vi "Build Dqmh Module Relationship Graph.vi"(4 "Used Requests With Reply":T1[](array[typedef]), 6 "Request With Reply Links Info":T2[](array[typedef]), 7 "Module Name":string, 8 "Used Requests":T1[](array[typedef]), 9 "Registred Broadcast":T3[](array[typedef]), 10 "Broadcas Links Info":T2[](array[typedef]), 11 "Request Links Info":T2[](array[typedef])) -> (3 "Graph":string)   [LabVIEW 2021, in "TAF Proj Document Type.lvlib" / "Dqmh Module.lvclass"]
uses:
  <vilib>/Wovalab/AntiDoc/Document Type/Add-ons/LabVIEW TAF Project/Dqmh Module/Dqmh Module.lvclass
  <vilib>/Wovalab/AntiDoc/Document Type/Add-ons/LabVIEW TAF Project/Dqmh Module/Event Callers--cluster.ctl
  <vilib>/Wovalab/AntiDoc/Document Type/Add-ons/LabVIEW TAF Project/Dqmh Module/Module Broadcast Registred--cluster.ctl
  <vilib>/Wovalab/AntiDoc/Document Type/Add-ons/LabVIEW TAF Project/Dqmh Module/Requests Used By Module--cluster.ctl
  <vilib>/Wovalab/AntiDoc/GraphBuilder/Renderer/Graphviz/Graphviz.lvclass
  C:/Program Files (x86)/National Instruments/LabVIEW 2021/vi.lib/Wovalab/AntiDoc/GraphBuilder/Renderer/Renderer.lvclass
  <vilib>/Wovalab/AntiDoc/GraphBuilder/Graph/Graph.lvclass
  <vilib>/Wovalab/AntiDoc/GraphBuilder/Shapes/Edge/Graphviz/Graphviz Edge Shape.lvclass
  <vilib>/Wovalab/AntiDoc/GraphBuilder/Shapes/Edge/Graphviz/Shape.ctl
  <vilib>/Wovalab/AntiDoc/GraphBuilder/Shapes/Edge/Graphviz/Colors.ctl
  <vilib>/Wovalab/AntiDoc/GraphBuilder/Shapes/Node/Graphviz/Colors.ctl
  <vilib>/Wovalab/AntiDoc/GraphBuilder/Shapes/Node/Graphviz/Shape.ctl
  <vilib>/Wovalab/AntiDoc/GraphBuilder/Renderer/Graphviz/Specific Node Shape Def.ctl
  <vilib>/Wovalab/AntiDoc/GraphBuilder/Shapes/Node/Graphviz/Graphviz Node Shape.lvclass
  <vilib>/Wovalab/AntiDoc/GraphBuilder/Node/Node.lvclass
  <vilib>/Wovalab/AntiDoc/Document Type/Add-ons/LabVIEW TAF Project/Dqmh Module/Link Type--enum.ctl
  <vilib>/Wovalab/AntiDoc/GraphBuilder/Renderer/Graphviz/Graph Direction.ctl
  <vilib>/Wovalab/AntiDoc/Document Type/Add-ons/LabVIEW TAF Project/TAF Proj Document Type.lvlib
  <vilib>/Wovalab/AntiDoc/Utilities/Utilities.lvlib
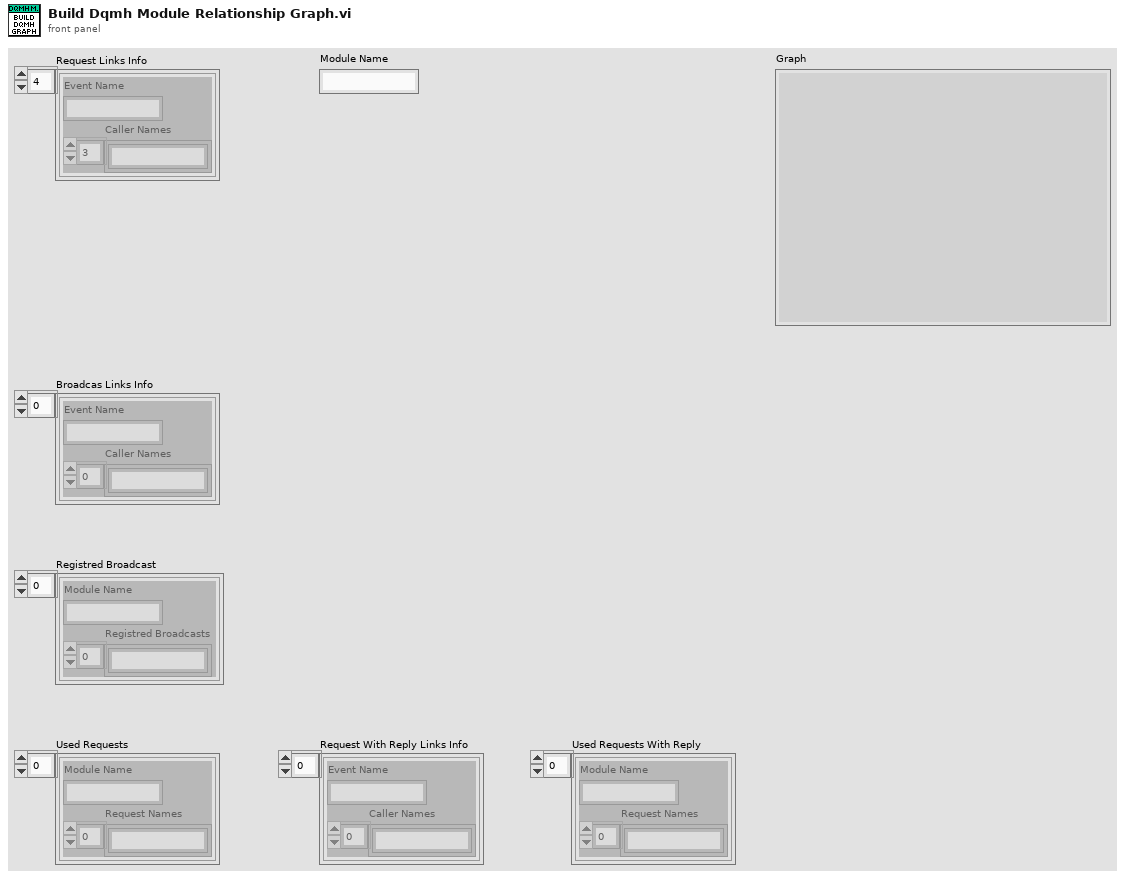
[diagram p1: front panel]
types:
  T1 = typedef "TAF Proj Document Type.lvlib/Dqmh Module.lvclass/Requests Used By Module--cluster.ctl" = cluster{"Module Name":string, "Request Names":string[]}
  T2 = typedef "TAF Proj Document Type.lvlib/Dqmh Module.lvclass/Event Callers--cluster.ctl" = cluster{"Event Name":string, "Caller Names":string[]}
  T3 = typedef "TAF Proj Document Type.lvlib/Dqmh Module.lvclass/Module Broadcast Registred--cluster.ctl" = cluster{"Module Name":string, "Registred Broadcasts":string[]}
  T4 = typedef "TAF Proj Document Type.lvlib/Dqmh Module.lvclass/Link Type--enum.ctl" = enum16{"Request", "Request With Reply", "Broadcast", "Registred Broadcast", "Used Requests", "Used Requests With Reply"}
  T5 = typedef "GraphBuilder.lvlib/Graphviz.lvclass/Graph Direction.ctl" = enum16{"Top to Bottom", "Left To Right", "Bottom to Top", "Right to Left"}
  T6 = typedef "GraphBuilder.lvlib/Graphviz Node Shape.lvclass/Colors.ctl" = enum16{"aliceblue", "antiquewhite", "aqua", "aquamarine", "azure", "beige", "bisque", "black", "blanchedalmond", "blue", "blueviolet", "brown", "burlywood", "cadetblue", "chartreuse", "chocolate", "coral", "cornflowerblue", "cornsilk", "crimson", "cyan", "darkblue", "darkcyan", "darkgoldenrod", "darkgray", "darkgreen", "darkgrey", "darkkhaki", "darkmagenta", "darkolivegreen", "darkorange", "darkorchid", "darkred", "darksalmon", "darkseagreen", "darkslateblue", "darkslategray", "darkslategrey", "darkturquoise", "darkviolet", "deeppink", "deepskyblue", "dimgray", "dimgrey", "dodgerblue", "firebrick", "floralwhite", "forestgreen", "fuchsia", "gainsboro", "ghostwhite", "gold", "goldenrod", "gray", "green", "greenyellow", "grey", "honeydew", "hotpink", "indianred", "indigo", "ivory", "khaki", "lavender", "lavenderblush", "lawngreen", "lemonchiffon", "lightblue", "lightcoral", "lightcyan", "lightgoldenrodyellow", "lightgray", "lightgreen", "lightgrey", "lightpink", "lightsalmon", "lightseagreen", "lightskyblue", "lightslategray", "lightslategrey", "lightsteelblue", "lightyellow", "lime", "limegreen", "linen", "magenta", "maroon", "mediumaquamarine", "mediumblue", "mediumorchid", "mediumpurple", "mediumseagreen", "mediumslateblue", "mediumspringgreen", "mediumturquoise", "mediumvioletred", "midnightblue", "mintcream", "mistyrose", "moccasin", "navajowhite", "navy", "oldlace", "olive", "olivedrab", "orange", "orangered", "orchid", "palegoldenrod", "palegreen", "paleturquoise", "palevioletred", "papayawhip", "peachpuff", "peru", "pink", "plum", "powderblue", "purple", "red", "rosybrown", "royalblue", "saddlebrown", "salmon", "sandybrown", "seagreen", "seashell", "sienna", "silver", "skyblue", "slateblue", "slategray", "slategrey", "snow", "springgreen", "steelblue", "tan", "teal", "thistle", "tomato", "turquoise", "violet", "wheat", "white", "whitesmoke", "yellow", "yellowgreen"}
  T7 = typedef "GraphBuilder.lvlib/Graphviz.lvclass/Specific Node Shape Def.ctl" = cluster{"Node ID":string, "Graphviz Node Shape":refnum<class "Graphviz Node Shape.lvclass">}
  T8 = typedef "GraphBuilder.lvlib/Graphviz Node Shape.lvclass/Shape.ctl" = enum16{"box", "polygon", "ellipse", "oval", "circle", "point", "egg", "triangle", "plaintext", "plain", "diamond", "trapezium", "parallelogram", "house", "pentagon", "hexagon", "septagon", "octagon", "doublecircle", "doubleoctagon", "tripleoctagon", "invtriangle", "invtrapezium", "invhouse", "Mdiamond", "Msquare", "Mcircle", "rect", "rectangle", "square", "star", "none", "underline", "cylinder", "note", "tab", "folder", "box3D", "component", "promoter", "cds", "terminator", "utr", "primersite", "restrictionsite", "fivepoverhang", "threepoverhang", "noverhang", "assembly", "signature", "insulator", "ribosite", "rnastab", "proteasesite", "proteinstab", "rpromoter", "rarrow", "larrow", "lpromoter"}
  T9 = typedef "GraphBuilder.lvlib/Graphviz Edge Shape.lvclass/Colors.ctl" = enum16{"aliceblue", "antiquewhite", "aqua", "aquamarine", "azure", "beige", "bisque", "black", "blanchedalmond", "blue", "blueviolet", "brown", "burlywood", "cadetblue", "chartreuse", "chocolate", "coral", "cornflowerblue", "cornsilk", "crimson", "cyan", "darkblue", "darkcyan", "darkgoldenrod", "darkgray", "darkgreen", "darkgrey", "darkkhaki", "darkmagenta", "darkolivegreen", "darkorange", "darkorchid", "darkred", "darksalmon", "darkseagreen", "darkslateblue", "darkslategray", "darkslategrey", "darkturquoise", "darkviolet", "deeppink", "deepskyblue", "dimgray", "dimgrey", "dodgerblue", "firebrick", "floralwhite", "forestgreen", "fuchsia", "gainsboro", "ghostwhite", "gold", "goldenrod", "gray", "green", "greenyellow", "grey", "honeydew", "hotpink", "indianred", "indigo", "ivory", "khaki", "lavender", "lavenderblush", "lawngreen", "lemonchiffon", "lightblue", "lightcoral", "lightcyan", "lightgoldenrodyellow", "lightgray", "lightgreen", "lightgrey", "lightpink", "lightsalmon", "lightseagreen", "lightskyblue", "lightslategray", "lightslategrey", "lightsteelblue", "lightyellow", "lime", "limegreen", "linen", "magenta", "maroon", "mediumaquamarine", "mediumblue", "mediumorchid", "mediumpurple", "mediumseagreen", "mediumslateblue", "mediumspringgreen", "mediumturquoise", "mediumvioletred", "midnightblue", "mintcream", "mistyrose", "moccasin", "navajowhite", "navy", "oldlace", "olive", "olivedrab", "orange", "orangered", "orchid", "palegoldenrod", "palegreen", "paleturquoise", "palevioletred", "papayawhip", "peachpuff", "peru", "pink", "plum", "powderblue", "purple", "red", "rosybrown", "royalblue", "saddlebrown", "salmon", "sandybrown", "seagreen", "seashell", "sienna", "silver", "skyblue", "slateblue", "slategray", "slategrey", "snow", "springgreen", "steelblue", "tan", "teal", "thistle", "tomato", "turquoise", "violet", "wheat", "white", "whitesmoke", "yellow", "yellowgreen"}
  T10 = typedef "GraphBuilder.lvlib/Graphviz Edge Shape.lvclass/Shape.ctl" = enum16{"box", "lbox", "rbox", "obox", "olbox", "orbox", "crow", "lcrow", "rcrow", "diamond", "ldiamond", "rdiamond", "odiamond", "oldiamond", "ordiamond", "dot", "odot", "inv", "linv", "rinv", "oinv", "olinv", "orinv", "none", "normal", "lnormal", "rnormal", "onormal", "olnormal", "ornormal", "tee", "ltee", "rtee", "vee", "lvee", "rvee", "curve", "lcurve", "rcurve", "icurve", "licurve", "ricurve"}
  T11 = typedef "GraphBuilder.lvlib/Graphviz.lvclass/Specific Edge Shape Def.ctl" = cluster{"Source Node ID":string, "Target Node ID":string, "Caption":string, "Graphviz Edge Shape":refnum<class "Graphviz Edge Shape.lvclass">}
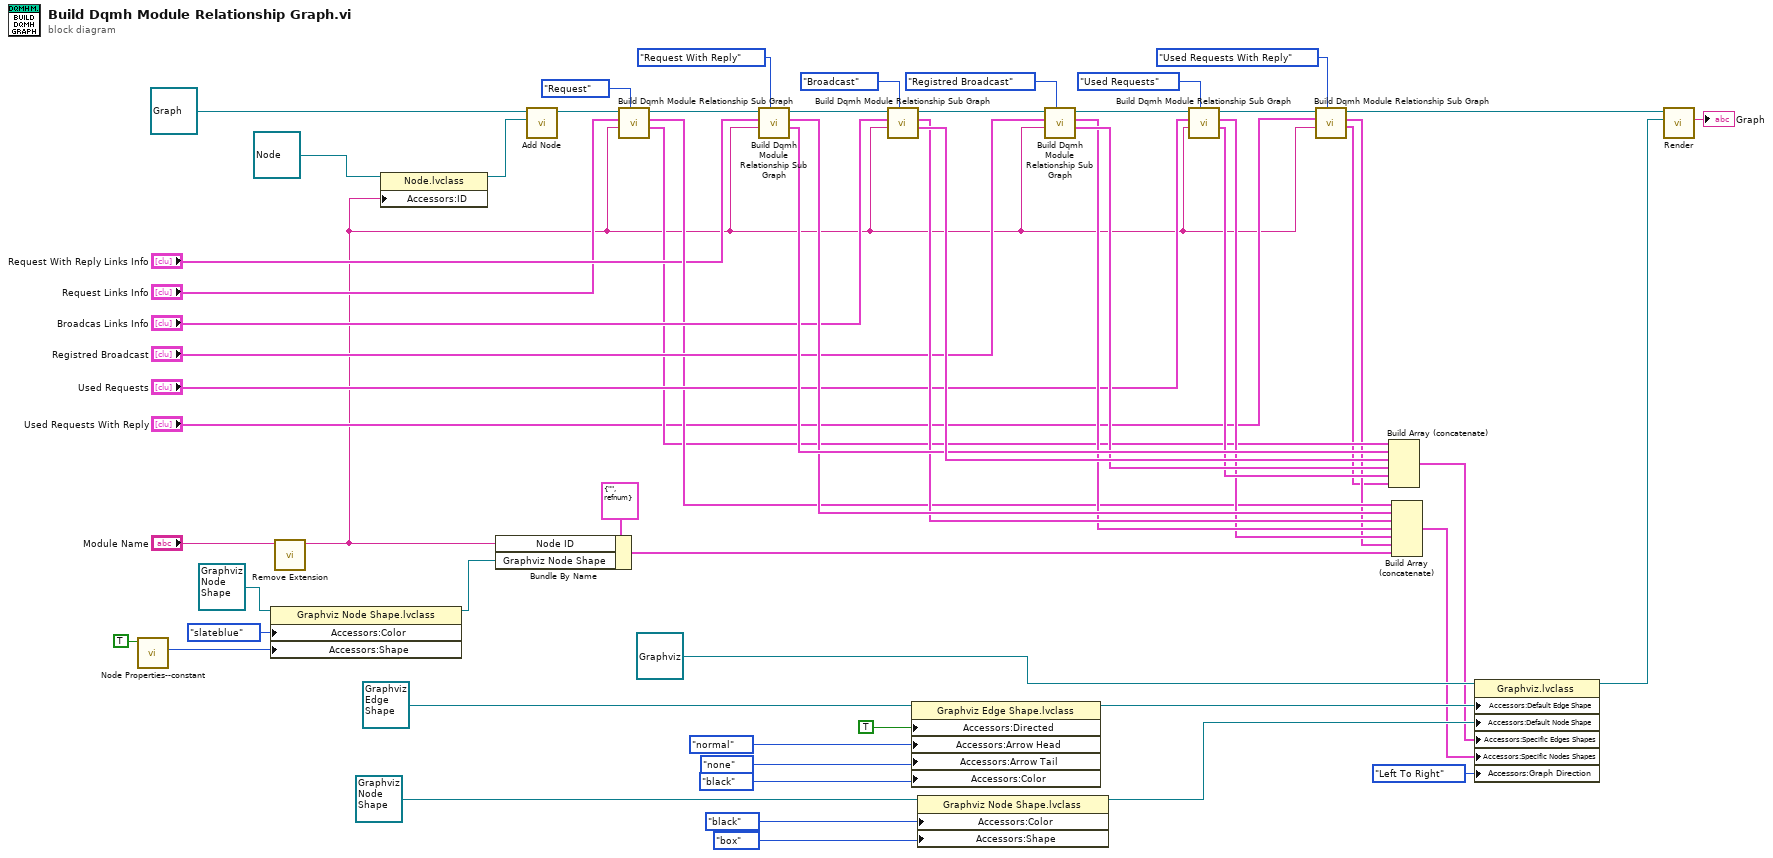
[diagram p0: block diagram]
diagram:
  n1 = call <vilib>:"Node Properties--constant.vi"("Lvlib"=TRUE) -> ("Shape"=w21:T8)  [unwired: 9 in, 1 out]
  n2 = property class="Graphviz Node Shape.lvclass"(reference=refnum<class "Graphviz Node Shape.lvclass"> refnum ("GraphBuilder.lvlib:Graphviz Node Shape.lvclass"), "Accessors:Color"=Colors."slateblue" ("Color"), "Accessors:Shape"=w21) -> (reference out=w40:refnum<class "Graphviz Node Shape.lvclass">)  [unwired: 1 in, 1 out]
  n3 = call <vilib>:"Remove Extension.vi"("File Name"="Module Name") -> ("File Name Without Extension"=w1:string)  [unwired: 10 in]
  n4 = property class="Node.lvclass"(reference=refnum<class "Node.lvclass"> refnum ("GraphBuilder.lvlib:Node.lvclass"), "Accessors:ID"=w1) -> (reference out=w43:refnum<class "Node.lvclass">)  [unwired: 1 in, 1 out]
  n5 = Bundle By Name(cluster=T7 {"Node ID"="", "Graphviz Node Shape"=refnum} ("Specific Node Shape"), "Node ID"=w1, "Graphviz Node Shape"=w40) -> (w45:T7)
  n6 = call-dynamic "Add Node.vi"("Node"=w43, "Graph in"=refnum<class "Graph.lvclass"> refnum ("GraphBuilder.lvlib:Graph.lvclass")) -> ("Graph out"=w14:refnum<class "Graph.lvclass">)  [unwired: 8 in, 1 out]
  n7 = call <vilib>:"Build Dqmh Module Relationship Sub Graph.vi"("Link Type"=Link_Type--enum."Request", "Module Name"=w1, "Links Info"="Request Links Info", "Graph in"=w14) -> ("Specific Edge Shape"=w9:T11[], "Specific Node Shape"=w12:T7[], "Graph out"=w13:refnum<class "Graph.lvclass">)  [unwired: 5 in]
  n8 = call <vilib>:"Build Dqmh Module Relationship Sub Graph.vi"("Link Type"=Link_Type--enum."Request With Reply", "Module Name"=w1, "Links Info"="Request With Reply Links Info", "Graph in"=w13) -> ("Specific Edge Shape"=w36:T11[], "Specific Node Shape"=w34:T7[], "Graph out"=w38:refnum<class "Graph.lvclass">)  [unwired: 5 in]
  n9 = call <vilib>:"Build Dqmh Module Relationship Sub Graph.vi"("Link Type"=Link_Type--enum."Broadcast", "Module Name"=w1, "Links Info"="Broadcas Links Info", "Graph in"=w38) -> ("Specific Edge Shape"=w37:T11[], "Specific Node Shape"=w33:T7[], "Graph out"=w29:refnum<class "Graph.lvclass">)  [unwired: 5 in]
  n10 = property class="Graphviz Edge Shape.lvclass"(reference=refnum<class "Graphviz Edge Shape.lvclass"> refnum ("GraphBuilder.lvlib:Graphviz Edge Shape.lvclass"), "Accessors:Directed"=TRUE ("Directed"), "Accessors:Arrow Head"=Shape."normal" ("Arrow Head"), "Accessors:Arrow Tail"=Shape."none" ("Arrow Tail"), "Accessors:Color"=Colors."black" ("Color")) -> (reference out=w56:refnum<class "Graphviz Edge Shape.lvclass">)  [unwired: 1 in, 1 out]
  n11 = property class="Graphviz Node Shape.lvclass"(reference=refnum<class "Graphviz Node Shape.lvclass"> refnum ("GraphBuilder.lvlib:Graphviz Node Shape.lvclass"), "Accessors:Color"=Colors."black" ("Color"), "Accessors:Shape"=Shape."box" ("Shape")) -> (reference out=w57:refnum<class "Graphviz Node Shape.lvclass">)  [unwired: 1 in, 1 out]
  n12 = call <vilib>:"Build Dqmh Module Relationship Sub Graph.vi"("Link Type"=Link_Type--enum."Registred Broadcast", "Module Name"=w1, "Links Info"="Registred Broadcast", "Graph in"=w29) -> ("Specific Edge Shape"=w26:T11[], "Specific Node Shape"=w25:T7[], "Graph out"=w19:refnum<class "Graph.lvclass">)  [unwired: 5 in]
  n13 = call <vilib>:"Build Dqmh Module Relationship Sub Graph.vi"("Link Type"=Link_Type--enum."Used Requests", "Module Name"=w1, "Links Info"="Used Requests", "Graph in"=w19) -> ("Specific Edge Shape"=w17:T11[], "Specific Node Shape"=w16:T7[], "Graph out"=w7:refnum<class "Graph.lvclass">)  [unwired: 5 in]
  n14 = call <vilib>:"Build Dqmh Module Relationship Sub Graph.vi"("Link Type"=Link_Type--enum."Used Requests With Reply", "Module Name"=w1, "Links Info"="Used Requests With Reply", "Graph in"=w7) -> ("Specific Edge Shape"=w3:T11[], "Specific Node Shape"=w4:T7[], "Graph out"=w6:refnum<class "Graph.lvclass">)  [unwired: 5 in]
  n15 = Build Array (concatenate)(w9, w36, w37, w26, w17, w3) -> (w35:T11[])
  n16 = Build Array (concatenate)(w12, w34, w33, w25, w16, w4, w45) -> (w44:T7[])
  n17 = property class="Graphviz.lvclass"(reference=refnum<class "Graphviz.lvclass"> refnum ("GraphBuilder.lvlib:Graphviz.lvclass"), "Accessors:Default Edge Shape"=w56, "Accessors:Default Node Shape"=w57, "Accessors:Specific Edges Shapes"=w35, "Accessors:Specific Nodes Shapes"=w44, "Accessors:Graph Direction"=Graph_Direction."Left To Right" ("Graph Direction")) -> (reference out=w58:refnum<class "Graphviz.lvclass">)  [unwired: 1 in, 1 out]
  n18 = call-dynamic "Render.vi"("Renderer"=w58, "Graph in"=w6) -> ("Rendered Stream"=→"Graph":string)  [unwired: 7 in, 2 out]
